vi "Open Logging Settings from File.vi"(11 "Error In":errorcluster) -> (4 "Logging Settings":T1={"Logging Interval [s]"=1.0, "Use Lowpass Filter"=TRUE, "Tf [s]"=5.0, "Logging Data to File"=TRUE, "Log Folder"=path "c:/Temp/Data.lvm", "Logging Data to Cloud Service"=FALSE, "Data Cloud Service Url"="http://127.0.0.1:8001/DataWS", "Use Random Data"=TRUE}, 15 "Error Out":errorcluster)   [LabVIEW 2019]
uses:
  Controls/Logging Settings.ctl
  <vilib>/Utility/config.llb/Read Key (Double).vi
  <vilib>/Utility/config.llb/Read Key (Boolean).vi
  <vilib>/Utility/config.llb/Read Key (Path).vi
  <vilib>/Utility/config.llb/Read Key (String).vi
  <vilib>/Utility/config.llb/NI_LVConfig.lvlib
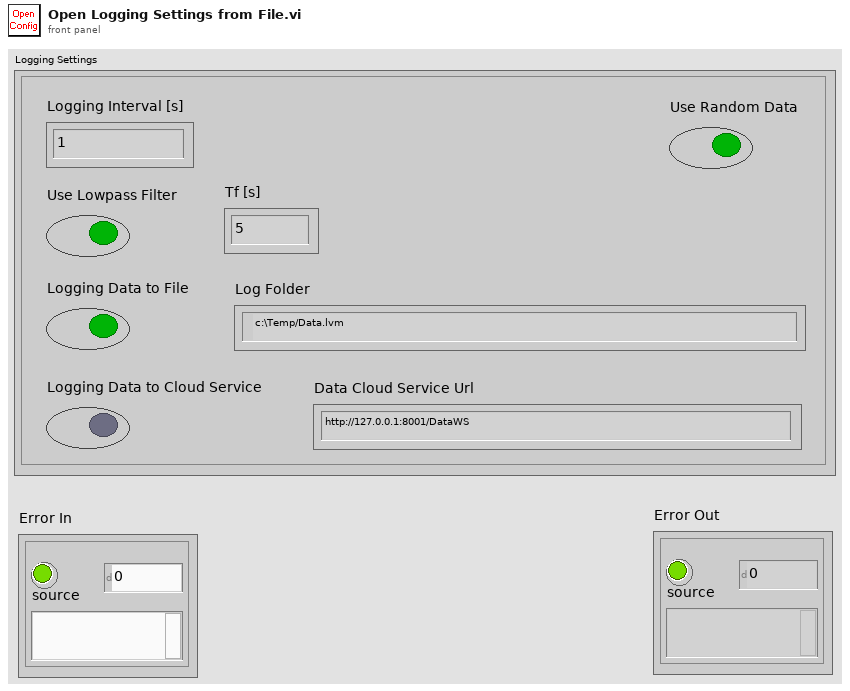
[diagram p1: front panel]
types:
  T1 = typedef "Logging Settings.ctl" = cluster{"Logging Interval [s]":dbl, "Use Lowpass Filter":bool, "Tf [s]":dbl, "Logging Data to File":bool, "Log Folder":path, "Logging Data to Cloud Service":bool, "Data Cloud Service Url":string, "Use Random Data":bool}
  T2 = typedef "NI_LVConfig.lvlib/Config Data RefNum.ctl" = refnum<k1>
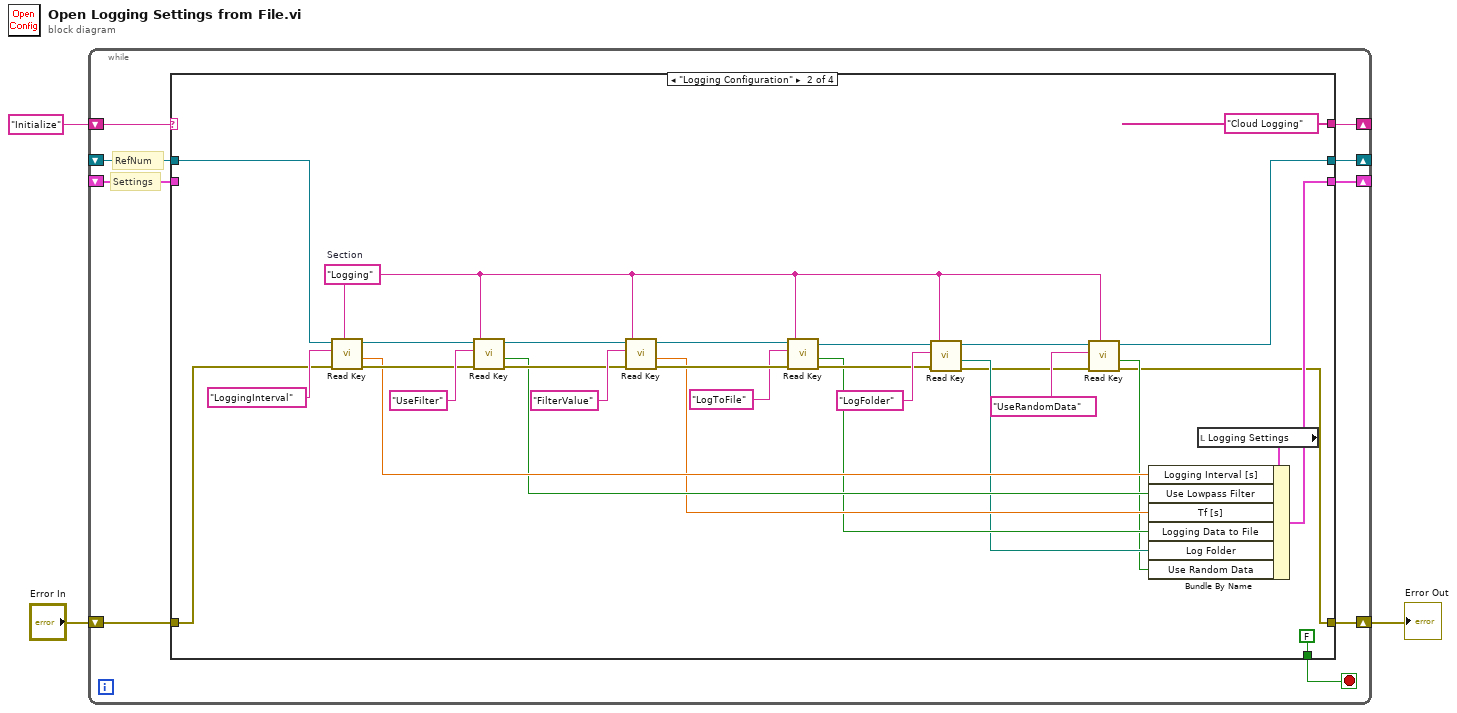
[diagram p0: block diagram]
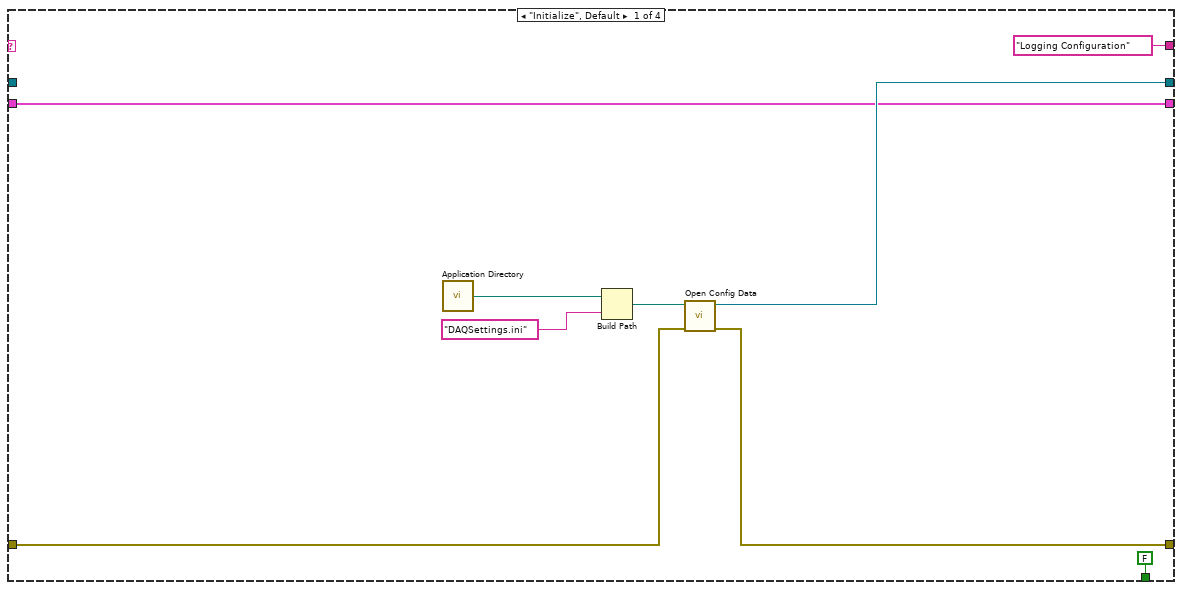
[diagram p2: hidden frame]
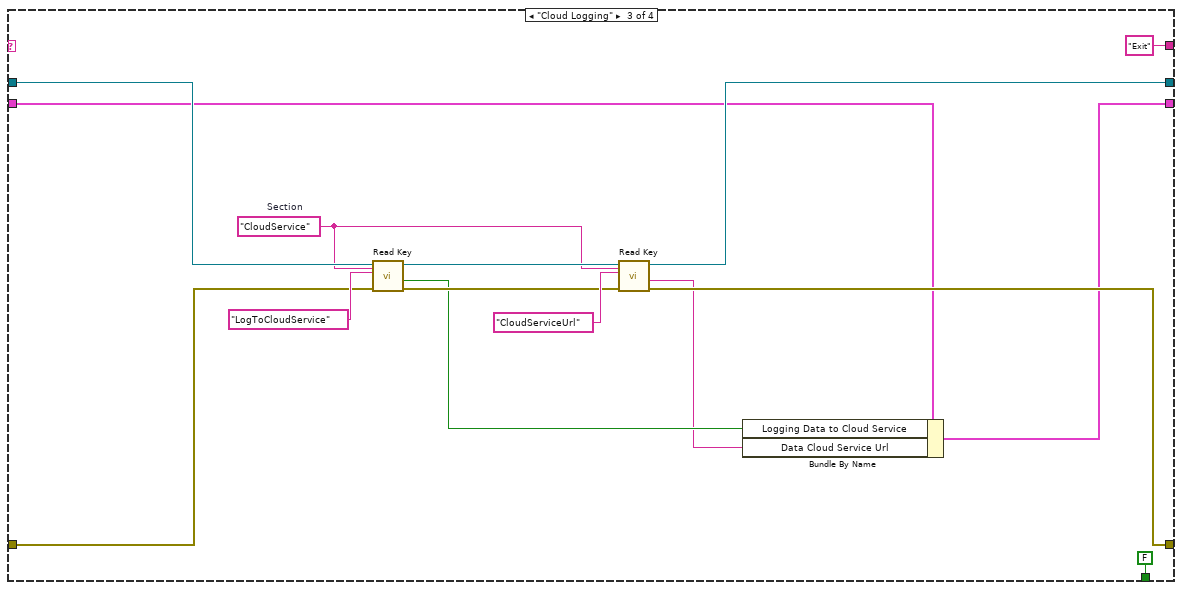
[diagram p3: hidden frame]
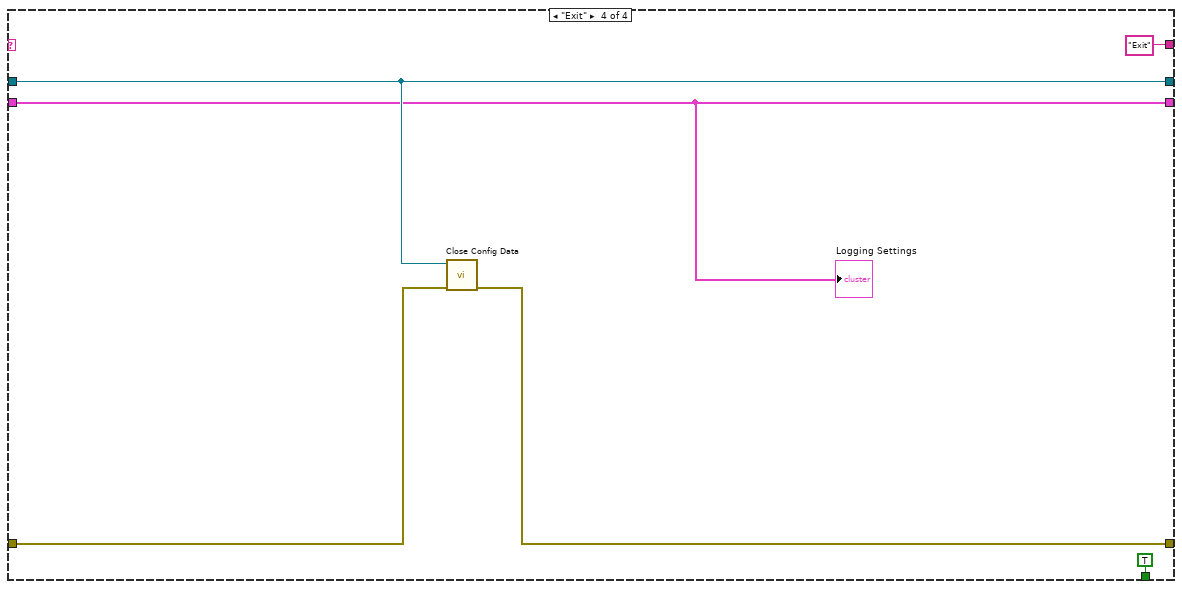
[diagram p4: hidden frame]
diagram:
  n1 = while {
    shift-right: [w7] -> _
    shift-left: "Initialize" ("key") -> [w12]
    shift-right: [w8] -> _
    shift-left: _ -> [w11]
    shift-right: [w9] -> w1
    shift-left: "Error In" -> [w10]
    shift-right: [w4] -> _
    shift-left: _ -> [w5]
    stop <- w6 stop-if-true
    # "Settings"
    # "RefNum"
    n2 = case shown="\"Logging Configuration\"" w12 {
      tunnel: w11 -> [_ w48 w63 w71]
      tunnel: w10 -> [w21 w47 w62 w73]
      tunnel: [w20 w22 w57 w72] -> w9
      tunnel: [w19 w23 w58 w71] -> w8
      tunnel: ["Logging Configuration" ("key") "Cloud Logging" ("key") "Exit" ("key") "Exit" ("key")] -> w7
      tunnel: [FALSE FALSE FALSE TRUE] -> w6
      tunnel: w5 -> [w13 _ w53 w68]
      tunnel: [w13 w29 w56 w68] -> w4
      frame "Initialize", Default {
        n3 = call <vilib>:"Application Directory.vi"() -> ("Application Directory"=w16:path)
        n4 = Build Path(base path=w16, name or relative path="DAQSettings.ini") -> (appended path=w14:path)
        n5 = call <vilib>:"Open Config Data.vi"("error in (no error)"=w21, "configuration file path"=w14) -> ("error out"=w20:errorcluster, "refnum"=w19:T2)  [unwired: 7 in, 1 out]
      }
      frame "Logging Configuration" {
        w26 = "Logging"  # Section
        n6 = call-poly <vilib>:"Read Key.vi"("section"=w26, "error in (no error)"=w47, "key"="LoggingInterval", "refnum"=w48) -> ("error out"=w51:errorcluster, "value"=w34:dbl, "refnum out"=w50:T2)  [unwired: 4 in, 1 out]
        n7 = call-poly <vilib>:"Read Key.vi"("section"=w26, "error in (no error)"=w51, "key"="UseFilter", "refnum"=w50) -> ("error out"=w42:errorcluster, "value"=w33:bool, "refnum out"=w43:T2)  [unwired: 4 in, 1 out]
        n8 = call-poly <vilib>:"Read Key.vi"("section"=w26, "error in (no error)"=w42, "key"="FilterValue", "refnum"=w43) -> ("error out"=w40:errorcluster, "value"=w32:dbl, "refnum out"=w41:T2)  [unwired: 4 in, 1 out]
        n9 = call-poly <vilib>:"Read Key.vi"("section"=w26, "error in (no error)"=w40, "key"="LogToFile", "refnum"=w41) -> ("error out"=w37:errorcluster, "value"=w31:bool, "refnum out"=w38:T2)  [unwired: 4 in, 1 out]
        n10 = call-poly <vilib>:"Read Key.vi"("section"=w26, "error in (no error)"=w37, "key"="LogFolder", "refnum"=w38) -> ("error out"=w25:errorcluster, "value"=w30:path, "refnum out"=w27:T2)  [unwired: 4 in, 1 out]
        n11 = call-poly <vilib>:"Read Key.vi"("section"=w26, "error in (no error)"=w25, "key"="UseRandomData", "refnum"=w27) -> ("error out"=w22:errorcluster, "value"=w24:bool, "refnum out"=w23:T2)  [unwired: 4 in, 1 out]
        n12 = local read "Logging Settings"() -> (w35:T1)
        n13 = Bundle By Name(cluster=w35, "Logging Interval [s]"=w34, "Use Lowpass Filter"=w33, "Tf [s]"=w32, "Logging Data to File"=w31, "Log Folder"=w30, "Use Random Data"=w24) -> (w29:T1)
      }
      frame "Cloud Logging" {
        w59 = "CloudService"  # Section
        n14 = call-poly <vilib>:"Read Key.vi"("section"=w59, "error in (no error)"=w62, "key"="LogToCloudService", "refnum"=w63) -> ("error out"=w66:errorcluster, "value"=w55:bool, "refnum out"=w65:T2)  [unwired: 4 in, 1 out]
        n15 = call-poly <vilib>:"Read Key.vi"("section"=w59, "error in (no error)"=w66, "key"="CloudServiceUrl", "refnum"=w65) -> ("error out"=w57:errorcluster, "value"=w54:string, "refnum out"=w58:T2)  [unwired: 4 in, 1 out]
        n16 = Bundle By Name(cluster=w53, "Logging Data to Cloud Service"=w55, "Data Cloud Service Url"=w54) -> (w56:T1)
      }
      frame "Exit" {
        n17 = call <vilib>:"Close Config Data.vi"("error in (no error)"=w73, "refnum"=w71) -> ("error out"=w72:errorcluster)  [unwired: 8 in, 1 out]
        "Logging Settings" <- w68
      }
    }
  }
  "Error Out" <- w1
